vi "JsonFile_SetAttribute(Path).vi"(8 "error in (no error)":errorcluster, 9 "Value":path, 10 "Attribute":string, 11 "Json":path) -> (0 "error out":errorcluster, 3 "Json (dup)":path)   [LabVIEW 2019, in "lv-apt-json-file.lvlib"]
uses:
  lv-apt-json-file.lvlib
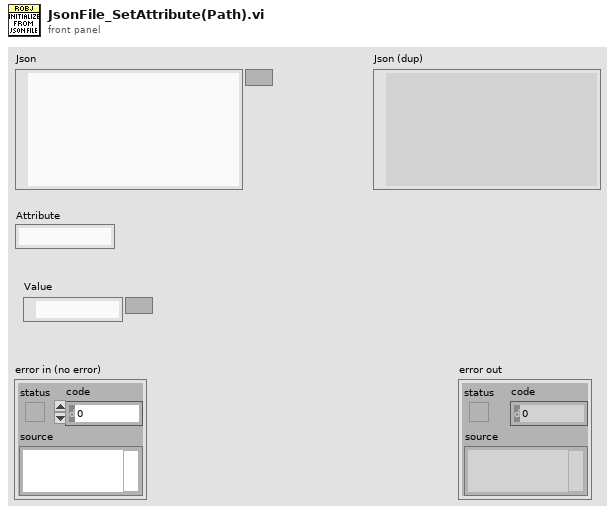
[diagram p1: front panel]
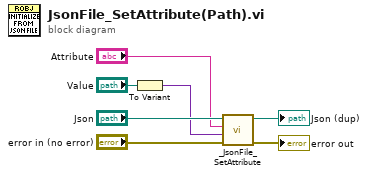
[diagram p0: block diagram]
diagram:
  n1 = To Variant(anything="Value") -> (Variant=w1:variant)
  n2 = call "_JsonFile_SetAttribute.vi"("error in (no error)"="error in (no error)", "Value"=w1, "Attribute"="Attribute", "Json"="Json") -> ("error out"=→"error out":errorcluster, "Json (dup)"=→"Json (dup)":path)  [unwired: 6 in]
